vi "Compute DistanceComplex.vi"   [LabVIEW 2011]
doc: "Using the camera lens information and the real world width of the target, determine the distance to the target."
types:
  T1 = cluster{"X Image Resolution":i32, "Y Image Resolution":i32}
  T2 = cluster{"X Image Resolution":dbl, "Y Image Resolution":dbl}
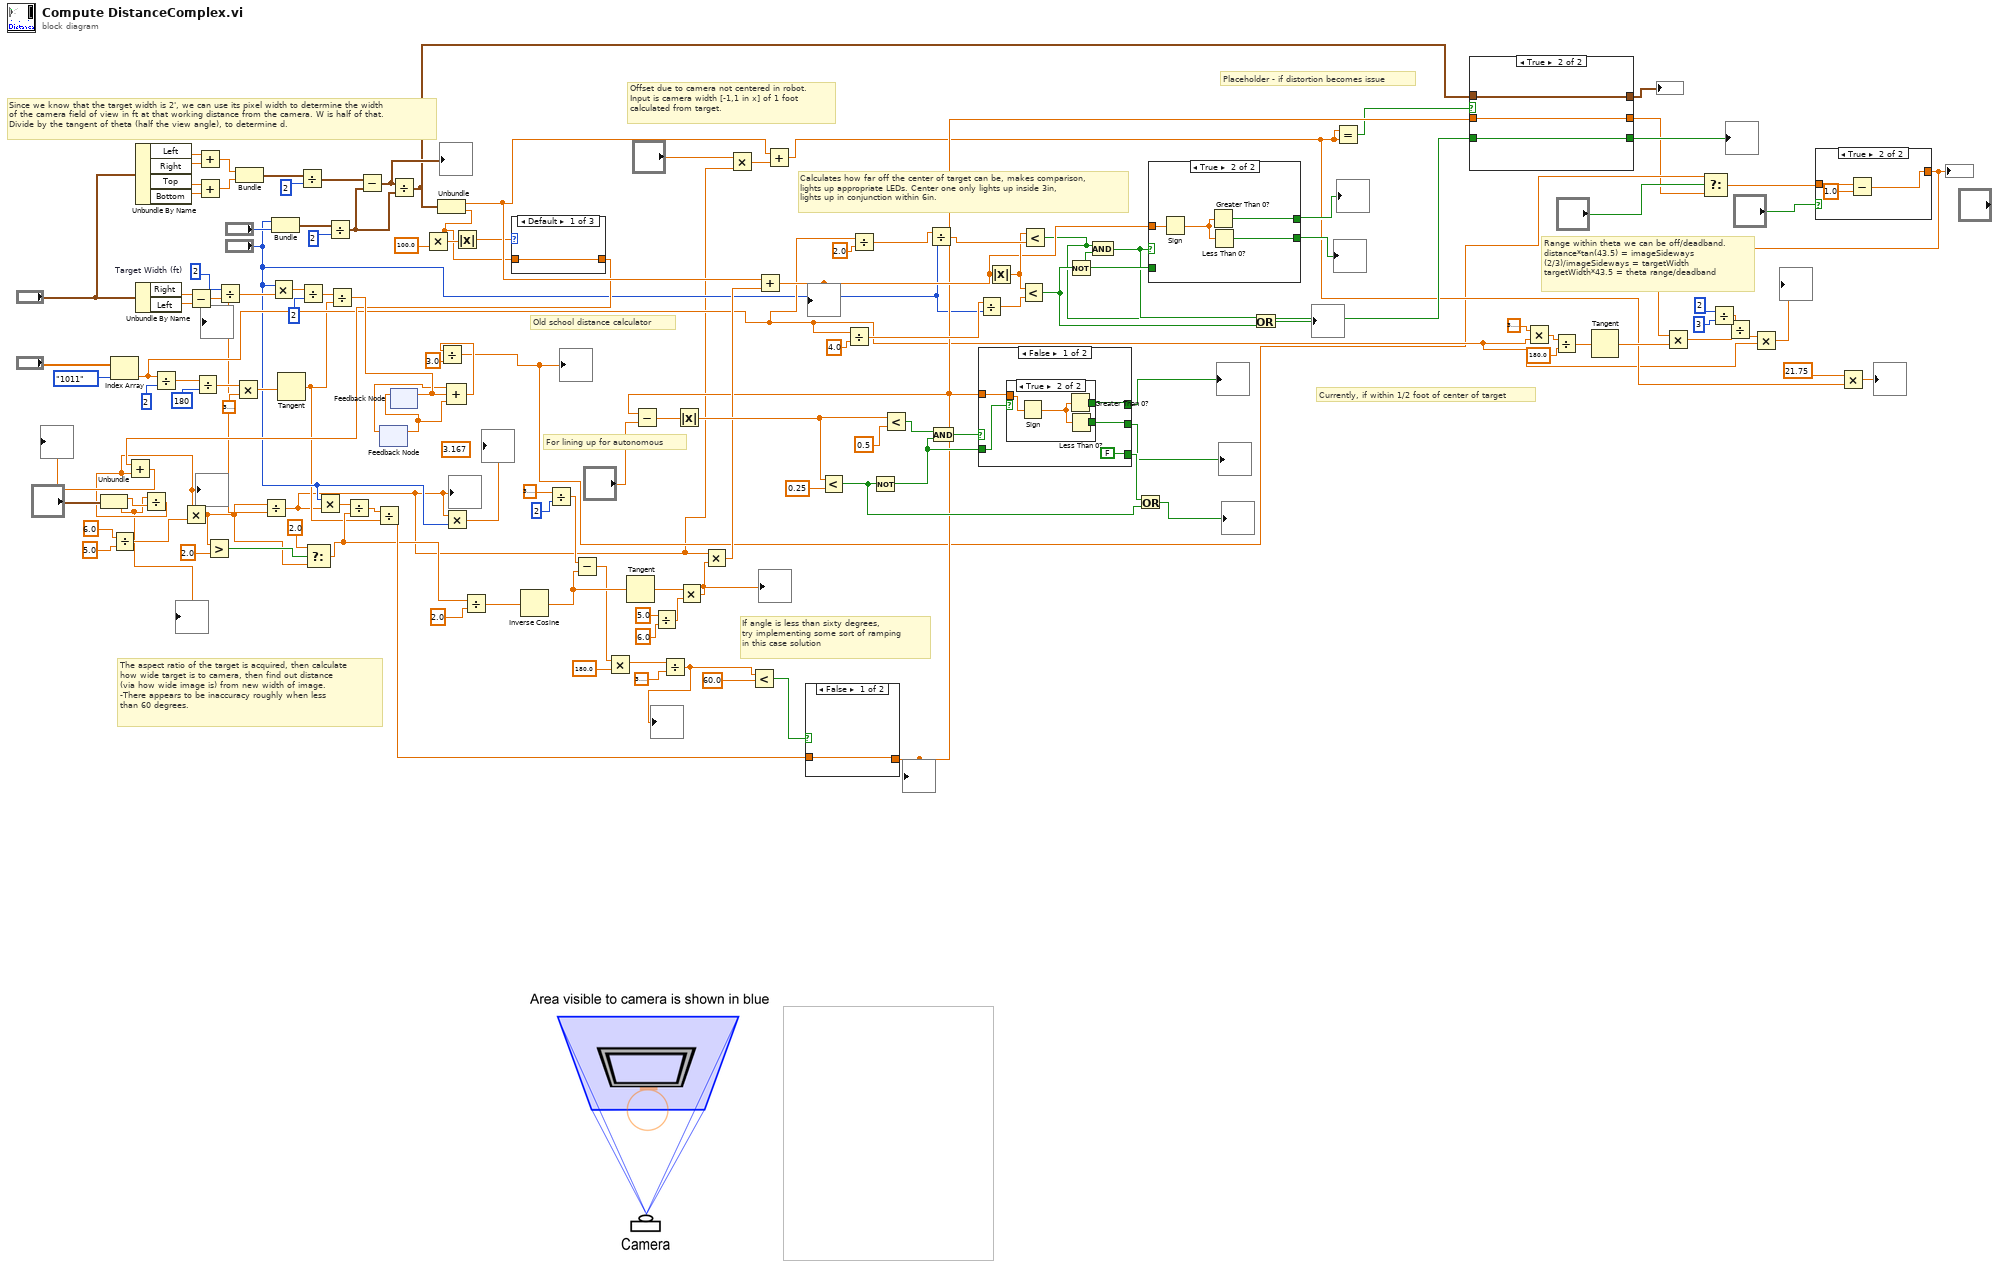
[diagram p0: block diagram]
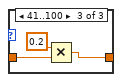
[diagram p4: hidden frame]
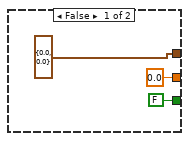
[diagram p5: hidden frame]
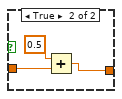
[diagram p6: hidden frame]
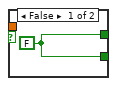
[diagram p7: hidden frame]
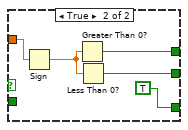
[diagram p8: hidden frame]
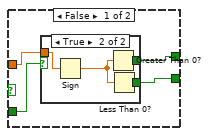
[diagram p9: hidden frame]
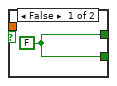
[diagram p10: hidden frame]
diagram:
  (unwired) 3.167 ("y")
  w126 = 2  # Target Width (ft)
  # "Offset due to camera not centered in robot.\nInput is camera width [-1,1 in x] of 1 foot \ncalculated from target."
  # "Range within theta we can be off/deadband.\ndistance*tan(43.5) = imageSideways\n(2/3)/imageSideways = targetWidth\ntargetWidth*43.5 = theta range/deadband"
  # "Placeholder - if distortion becomes issue"
  # "Currently, if within 1/2 foot of center of target"
  # "Calculates how far off the center of target can be, makes comparison,\nlights up appropriate LEDs. Center one only lights up inside 3in,\nlights up in conjunction within 6in."
  # "For lining up for autonomous"
  # "Old school distance calculator"
  # "The aspect ratio of the target is acquired, then calculate\nhow wide target is to camera, then find out distance \n(via how wide image is) from new width of image. \n-There appears to be inaccuracy roughly when less\nthan 60 degrees."
  # "If angle is less than sixty degrees,\ntry implementing some sort of ramping\nin this case solution"
  # "Since we know that the target width is 2', we can use its pixel width to determine the width\nof the camera field of view in ft at that working distance from the camera. W is half of that.\nDivide by the tangent of theta (half the view angle), to determine d."
  n1 = Unbundle("?") -> ("Avg. Horizontal"=w86:dbl, "Avg. Vertical"=w4:dbl)
  "?" <- w4
  n2 = Index Array(array="?", index=enum16{"206", "1011"}."1011" ("Camera Type")) -> (element=w13:dbl)
  n3 = Divide(x=6.0, y=5.0) -> (x/y=w80:dbl)
  n4 = Unbundle By Name("?") -> ("Left"=w121:dbl, "Right"=w122:dbl, "Top"=w124:dbl, "Bottom"=w123:dbl)
  n5 = Unbundle By Name("?") -> ("Right"=w84:dbl, "Left"=w83:dbl)
  n6 = Divide(x=w4, y=w86) -> (x/y=w14:dbl)
  "?" <- w14
  n7 = Divide(x=w13, y=2) -> (x/y=w133:dbl)
  n8 = Multiply(x=w14, y=w80) -> (x*y=w22:dbl)
  n9 = Subtract(x=w84, y=w83) -> (x-y=w3:dbl)
  "?" <- w3
  n10 = Divide(x=w133, y=180) -> (x/y=w132:dbl)
  n11 = Add(x=w121, y=w122) -> (x+y=w119:dbl)
  n12 = Add(x=w124, y=w123) -> (x+y=w118:dbl)
  n13 = Greater?(x=w22, y=2.0) -> (0:w24:bool)
  n14 = Divide(x=w126, y=w3) -> (x/y=w127:dbl)
  n15 = Multiply(x=w132, y=3.141592653589793) -> (x*y=w134:dbl)
  n16 = Bundle(w119, w118) -> (w37:cluster{dbl, dbl})  [unwired: 1 in]
  n17 = Divide(x=w22, y=w3) -> (x/y=w1:dbl)
  "?" <- w1
  n18 = Multiply(x="?", y=w127) -> (x*y=w128:dbl)
  n19 = Bundle("X Image Resolution"="?", "Y Image Resolution"="?") -> (w116:T1)  [unwired: 1 in]
  n20 = Tangent(1:w134) -> (0:w10:dbl)
  n21 = Divide(x=w37, y=2) -> (x/y=w36:cluster{dbl, dbl})
  n22 = Divide(x=w128, y=2) -> (x/y=w130:dbl)
  n23 = Select(t=2.0, s=w24, f=w22) -> (s? t:f=w21:dbl)
  n24 = Multiply(x="?", y=w1) -> (x*y=w64:dbl)
  n25 = Divide(x=w116, y=2) -> (x/y=w114:T2)
  n26 = Divide(x=w130, y=w10) -> (x/y=w113:dbl)
  n27 = Divide(x=w64, y=w21) -> (x/y=w85:dbl)
  n28 = Subtract(x=w36, y=w114) -> (x-y=w35:cluster{dbl, dbl})
  "?" <- w35
  n29 = Divide(x=w85, y=w10) -> (x/y=w56:dbl)
  n30 = feedback #1() -> (w32:dbl)  [unwired: 1 in]
  n31 = Divide(x=w35, y=w114) -> (x/y=w29:cluster{dbl, dbl})
  n32 = feedback #2() -> (w31:dbl)  [unwired: 1 in]
  n33 = feedback-in #1(w31) -> ()
  n34 = feedback-in #2(w113) -> ()
  n35 = Unbundle(w29) -> (w27:dbl, w16:dbl)
  n36 = Multiply(x=w16, y=100.0) -> (x*y=w18:dbl)
  n37 = Multiply(x=w1, y="?") -> (x*y=→"?":dbl)
  n38 = Compound Arithmetic op=ADD(w32, w113, w31) -> (w33:dbl)
  n39 = Divide(x=w33, y=3.0) -> (x/y=w8:dbl)
  "?" <- w8
  n40 = Absolute Value(x=w18) -> (abs(x)=w17:dbl)
  n41 = Divide(x=w21, y=2.0 ("x")) -> (x/y=w77:dbl)
  n42 = case shown="Default" w17 {
    tunnel: w16 -> [w138 w139 w142]
    tunnel: [w138 w139 w140] -> w15
    frame Default {
    }
    frame 0..40 {
    }
    frame 41..100 {
      n43 = Multiply(x=0.2, y=w142) -> (x*y=w140:dbl)
    }
  }
  n44 = Add(x=w15, y=w14) -> (x+y=→"?":dbl)
  n45 = Inverse Cosine(1:w77) -> (0:w71:dbl)
  n46 = Divide(x=3.141592653589793, y=2) -> (x/y=w76:dbl)
  n47 = Subtract(x=w76, y=w71) -> (x-y=w65:dbl)
  n48 = Multiply(x=w65, y=180.0) -> (x*y=w66:dbl)
  n49 = Tangent(1:w71) -> (0:w70:dbl)
  n50 = Divide(x=5.0, y=6.0) -> (x/y=w74:dbl)
  n51 = Divide(x=w66, y=3.141592653589793) -> (x/y=w59:dbl)
  "?" <- w59
  n52 = Multiply(x=w70, y=w74) -> (x*y=w62:dbl)
  "?" <- w62
  n53 = Multiply(x=w1, y=w62) -> (x*y=w61:dbl)
  n54 = Multiply(x="?", y=w1) -> (x*y=w28:dbl)
  n55 = Less?(x=w59, y=60.0) -> (x < y?=w57:bool)
  n56 = Add(x=w27, y=w61) -> (x+y=w63:dbl)
  "?" <- w63
  n57 = Add(x=w27, y=w28) -> (x+y=w26:dbl)
  n58 = case shown="False" w57 {
    tunnel: w56 -> [w143 w146]
    tunnel: [w143 w144] -> w54
    frame False {
    }
    frame True {
      n59 = Add(x=0.5, y=w146) -> (x+y=w144:dbl)
    }
  }
  "?" <- w54
  n60 = Subtract(x=w54, y="?") -> (x-y=w106:dbl)
  n61 = Absolute Value(x=w106) -> (abs(x)=w108:dbl)
  n62 = Less?(x=w108, y=0.25) -> (x < y?=w112:bool)
  n63 = Divide(x=w13, y=4.0) -> (x/y=w100:dbl)
  n64 = Divide(x=w13, y=2.0) -> (x/y=w102:dbl)
  n65 = Not(x=w112) -> (.not. x?=w98:bool)
  n66 = Less?(x=w108, y=0.5) -> (x < y?=w110:bool)
  n67 = Divide(x=w102, y="?") -> (x/y=w103:dbl)
  n68 = And(x=w110, y=w98) -> (x .and. y?=w92:bool)
  n69 = Divide(x=w100, y="?") -> (x/y=w88:dbl)
  n70 = case shown="False" w92 {
    tunnel: [w150 w160] -> w90
    tunnel: [w149 w159] -> w91
    tunnel: w54 -> [w151 w158]
    tunnel: w98 -> [w148 _]
    tunnel: [FALSE TRUE] -> w105
    frame False {
      n71 = case shown="True" w148 {
        tunnel: [w152 w155] -> w150
        tunnel: w151 -> [_ w154]
        tunnel: [w152 w153] -> w149
        frame False {
          w152 = FALSE
        }
        frame True {
          n72 = Sign(1:w154) -> (0:w156:dbl)
          n73 = Greater Than 0?(x=w156) -> (x > 0?=w155:bool)
          n74 = Less Than 0?(x=w156) -> (x < 0?=w153:bool)
        }
      }
    }
    frame True {
      n75 = Sign(1:w158) -> (0:w161:dbl)
      n76 = Greater Than 0?(x=w161) -> (x > 0?=w160:bool)
      n77 = Less Than 0?(x=w161) -> (x < 0?=w159:bool)
    }
  }
  "?" <- w91
  "?" <- w90
  n78 = Absolute Value(x=w63) -> (abs(x)=w89:dbl)
  n79 = Less?(x=w89, y=w88) -> (x < y?=w96:bool)
  n80 = Less?(x=w89, y=w103) -> (x < y?=w53:bool)
  n81 = Not(x=w96) -> (.not. x?=w97:bool)
  n82 = And(x=w53, y=w97) -> (x .and. y?=w60:bool)
  n83 = Or(x=w105, y=w112) -> (x .or. y?=→"?":bool)
  n84 = case shown="True" w60 {
    tunnel: w63 -> [w163 w174]
    tunnel: [w164 w172] -> w93
    tunnel: [w162 w171] -> w94
    tunnel: w97 -> [w165 _]
    frame False {
      n85 = case shown="True" w165 {
        tunnel: [w166 w169] -> w164
        tunnel: w163 -> [_ w168]
        tunnel: [w166 w167] -> w162
        frame False {
          w166 = FALSE
        }
        frame True {
          n86 = Sign(1:w168) -> (0:w170:dbl)
          n87 = Greater Than 0?(x=w170) -> (x > 0?=w169:bool)
          n88 = Less Than 0?(x=w170) -> (x < 0?=w167:bool)
        }
      }
    }
    frame True {
      n89 = Sign(1:w174) -> (0:w173:dbl)
      n90 = Greater Than 0?(x=w173) -> (x > 0?=w172:bool)
      n91 = Less Than 0?(x=w173) -> (x < 0?=w171:bool)
    }
  }
  "?" <- w94
  "?" <- w93
  n92 = Or(x=w60, y=w96) -> (x .or. y?=→"?":bool)
  n93 = Equal?(x=w26, y=w26) -> (x = y?=w51:bool)
  n94 = case shown="True" w51 {
    tunnel: w53 -> [_ w178]
    tunnel: w54 -> [_ w179]
    tunnel: w29 -> [_ w180]
    tunnel: [cluster{dbl, dbl} {0.0, 0.0} w180] -> w55
    tunnel: [0.0 w179] -> w7
    tunnel: [FALSE w178] -> w52
    frame False {
    }
    frame True {
    }
  }
  "?" <- w55
  "?" <- w52
  n95 = Multiply(x=3.141592653589793, y=w13) -> (x*y=w49:dbl)
  n96 = Divide(x=w49, y=180.0) -> (x/y=w47:dbl)
  n97 = Tangent(1:w47) -> (0:w44:dbl)
  n98 = Select(t=w8, s="?", f=w7) -> (s? t:f=w6:dbl)
  n99 = Divide(x=2, y=3) -> (x/y=w45:dbl)
  n100 = case shown="True" "?" {
    tunnel: w6 -> [w181 w184]
    tunnel: [w181 w182] -> w2
    frame False {
    }
    frame True {
      n101 = Subtract(x=w184, y=1.0) -> (x-y=w182:dbl)
    }
  }
  "?" <- w2
  n102 = Multiply(x=w2, y=w44) -> (x*y=w43:dbl)
  n103 = Divide(x=w45, y=w43) -> (x/y=w41:dbl)
  n104 = Multiply(x=w41, y=w13) -> (x*y=→"?":dbl)
  n105 = Multiply(x=21.75, y=w26) -> (x*y=→"?":dbl)
